vi "Release Client Message Queues.vi"(8 "error in (no error)":errorcluster, 11 "Client Message Queues":T1) -> (0 "error out":errorcluster)   [LabVIEW 2024, in "Message Queue.lvlib"]
doc: "Releases the message queues of the client."
uses:
  Message Queue.lvlib
  Client Message Queues.ctl
  Message Cluster.ctl
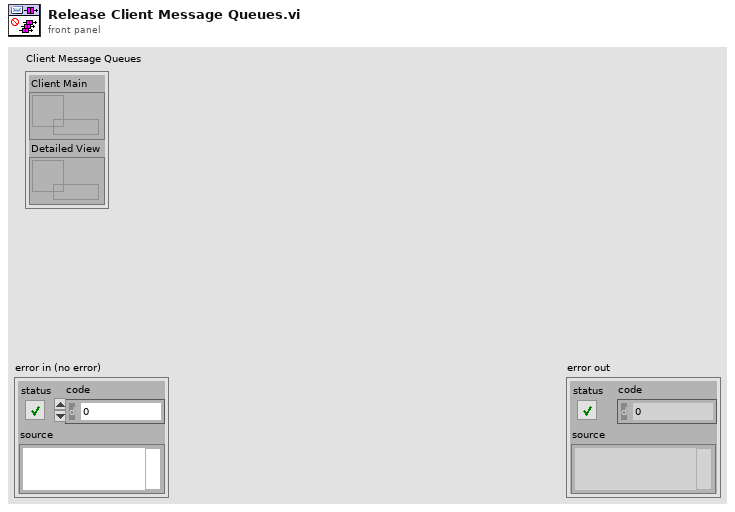
[diagram p1: front panel]
types:
  T1 = typedef "Message Queue.lvlib/Client Message Queues.ctl" = cluster{"Client Main":refnum<queue>, "Detailed View":refnum<queue>}
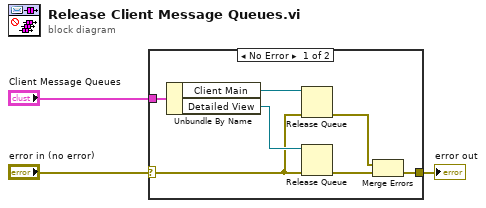
[diagram p0: block diagram]
diagram:
  n1 = case shown="No Error" "error in (no error)" {
    selector: "error in (no error)" -> [w4 w11]
    tunnel: [w7 w11] -> w3
    tunnel: "Client Message Queues" -> [w10 _]
    frame No Error {
      n2 = Unbundle By Name(w10) -> ("Client Main"=w9:refnum<queue>, "Detailed View"=w8:refnum<queue>)
      n3 = Release Queue(queue=w9, error in (no error)=w4) -> (error out=w6:errorcluster)  [unwired: 1 in, 2 out]
      n4 = Release Queue(queue=w8, error in (no error)=w4) -> (error out=w5:errorcluster)  [unwired: 1 in, 2 out]
      n5 = Merge Errors(w6, w5) -> (w7:errorcluster)
    }
    frame Error {
    }
  }
  "error out" <- w3
